vi "PFG600 5Byte checksum.vi"(1 "Input":string) -> (0 "Output":string)   [LabVIEW 2023]
panel:
  out "XOR":u8
  out "unsigned byte array":u8[](array[numeric])
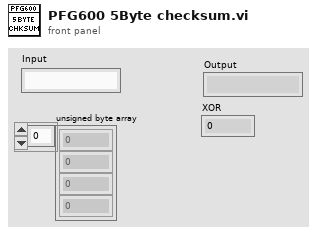
[diagram p1: front panel]
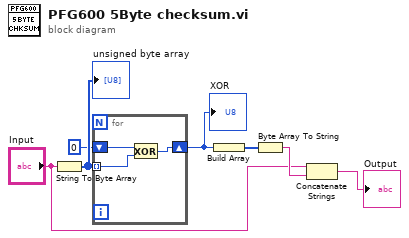
[diagram p0: block diagram]
diagram:
  n1 = String To Byte Array(string="Input") -> (unsigned byte array=w7:u8[])
  "unsigned byte array" <- w7
  n2 = for {
    tunnel: w7 -> [w10] mode=indexing
    shift-right: [w8] -> w4
    shift-left: u8 0 ("x") -> [w9]
    n3 = Exclusive Or(1:w10, 2:w9) -> (0:w8:u8)
  }
  "XOR" <- w4
  n4 = Build Array(w4) -> (w5:u8[])
  n5 = Byte Array To String(unsigned byte array=w5) -> (string=w3:string)
  n6 = Concatenate Strings("Input", w3) -> (→"Output":string)
